vi "XControl Test.vi"() -> ()   [LabVIEW 2011]
uses:
  Custom Combo Box.xctl
panel:
  out "Custom Combo Box":cluster{"String":string, "Value":string}[](xcontrol)
  in  "stop 2":bool
  out "data":string
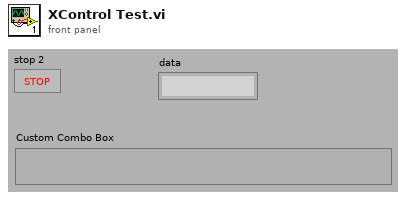
[diagram p1: front panel]
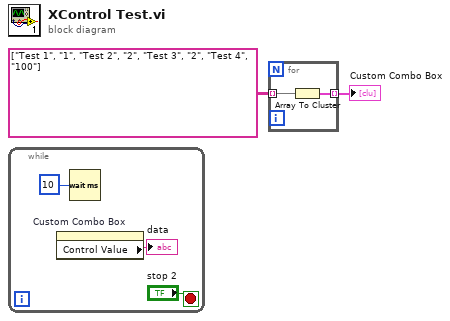
[diagram p0: block diagram]
diagram:
  n1 = while {
    stop <- "stop 2" stop-if-true
    n2 = property on="Custom Combo Box" class="Custom Combo Box (严格)"() -> ("Control Value"=→"data":string)  [unwired: 2 in, 2 out]
    n3 = Wait (ms)(milliseconds to wait=u32 10) -> ()  [unwired: 1 out]
  }
  n4 = for {
    tunnel: string[][] [["Test 1", "1"], ["Test 2", "2"], ["Test 3", "2"], ["Test 4", "100"]] -> [w7] mode=indexing
    tunnel: [w6] -> w1 mode=indexing
    n5 = Array To Cluster(array=w7) -> (cluster=w6:cluster{"[0]":string, "[1]":string})
  }
  "Custom Combo Box" <- w1
